vi "Trigger the captured image.vi"() -> ()   [LabVIEW 2018]
uses:
  LabViewDVPCamera/LabViewDVPCamera.lvlib
  <vilib>/picture/picture.llb/imagedata.ctl
panel:
  in  "image data":T1 caption="图像数据"
  in  "Trigger":bool
  in  "CloseFlg":i32
  out "handle":u32
  out "new picture":picture caption="新图片"
  in  "CameraList":u16(ring) items=["MGS130M-192.168.0.251"]
  in  "Set":bool
  in  "Close":bool
  in  "Open":bool
  in  "ScanCamera":bool
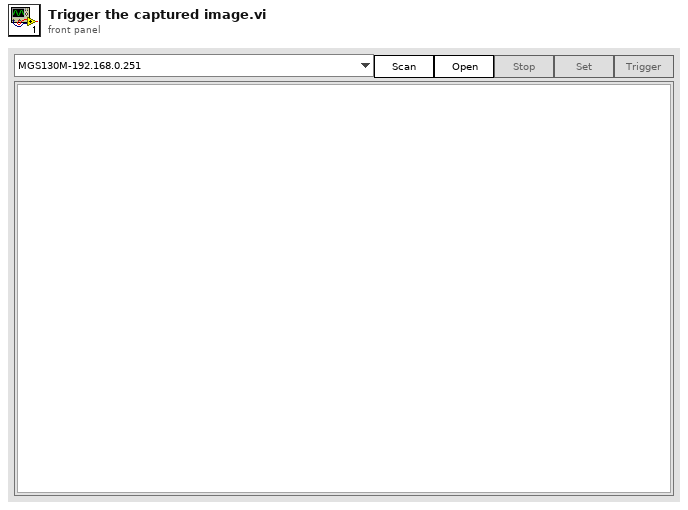
[diagram p1: front panel]
types:
  T1 = typedef "imagedata.ctl" = cluster{"image type":i32, "image depth":i32, "image":u8[], "mask":u8[], "colors":u32[], "Rectangle":cluster{"left":i16, "top":i16, "right":i16, "bottom":i16}}
  T2 = enum8{"Enabled", "Disabled", "Disabled and Grayed Out"}
  T3 = typedef "LVStringsAndValuesArrayTypeDef_U16.ctl" = cluster{"String":string, "Value":u16}[]
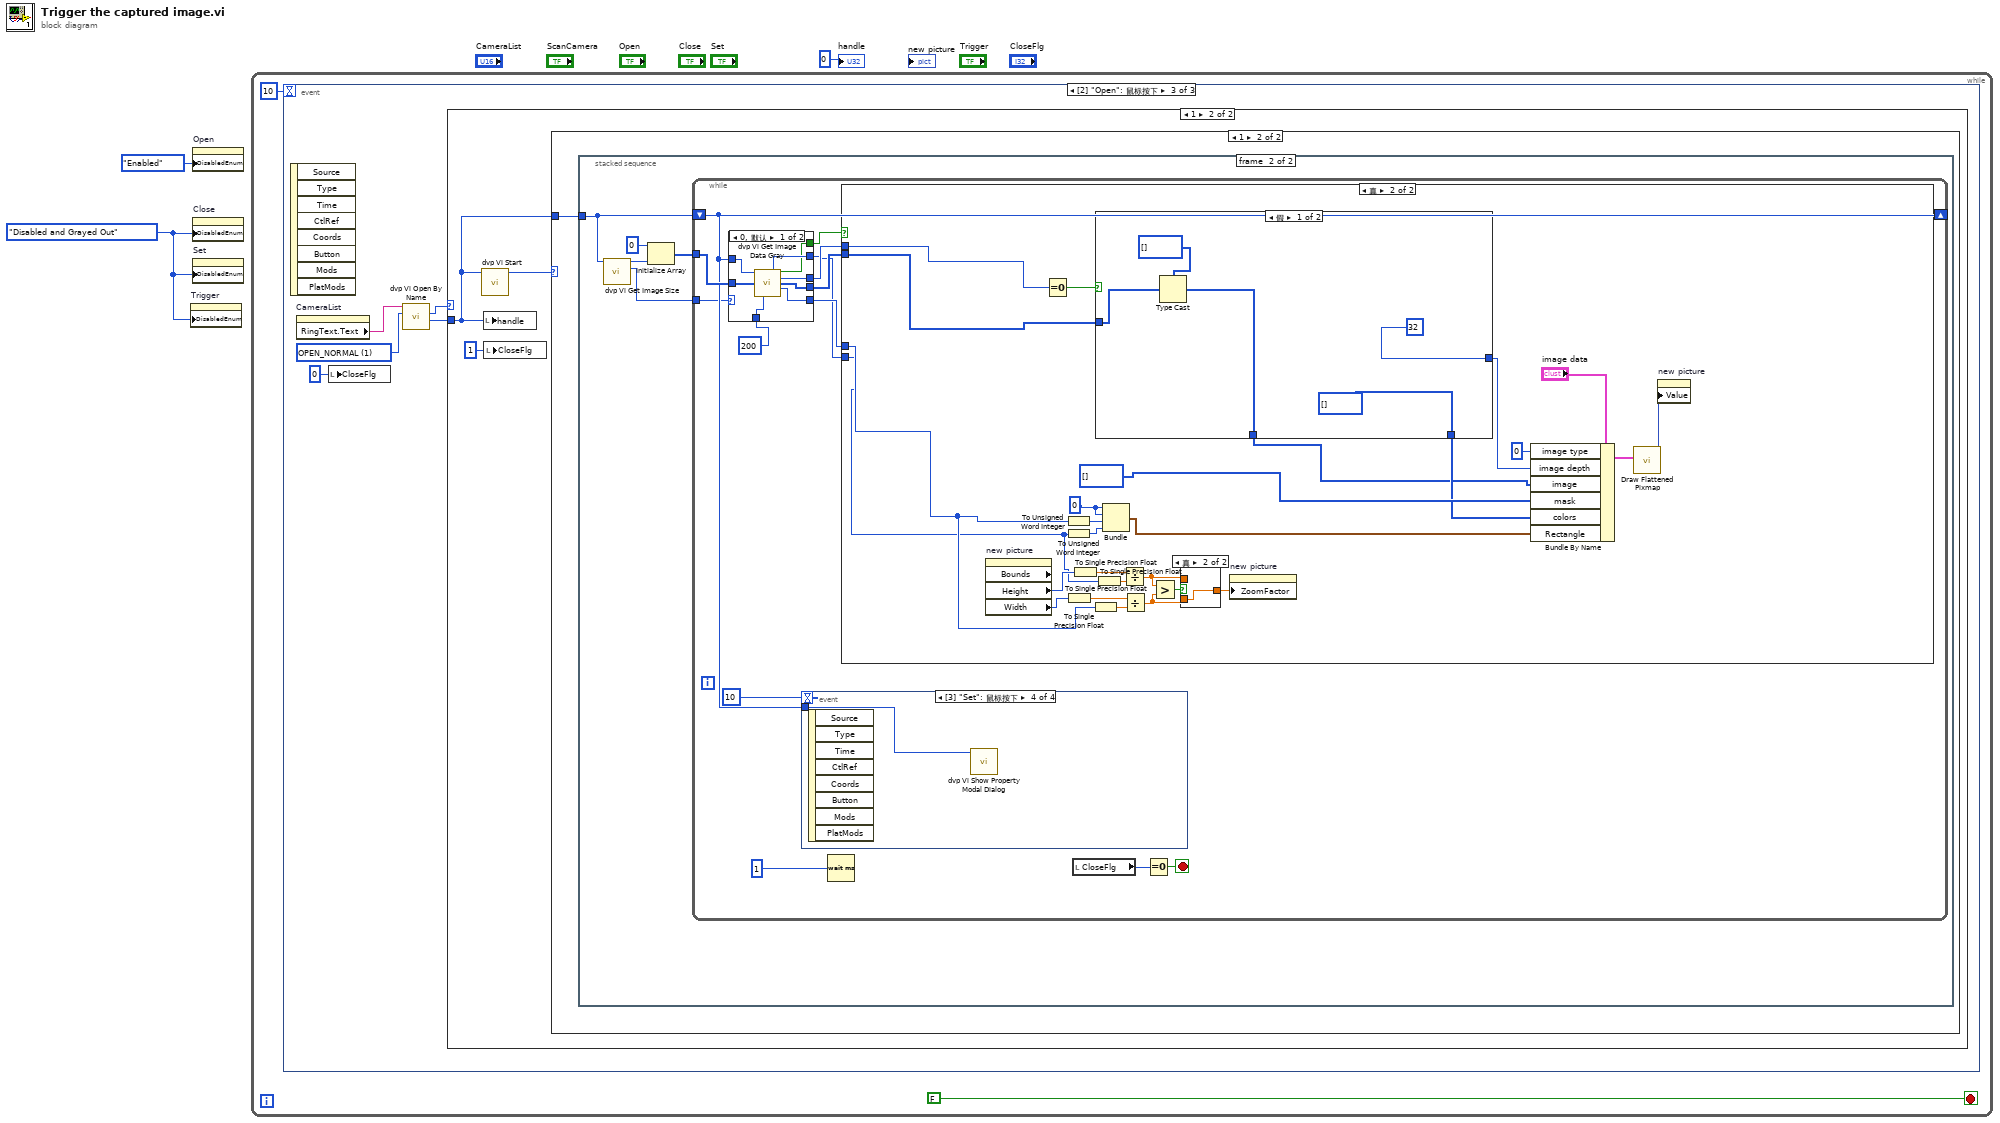
[diagram p0: block diagram]
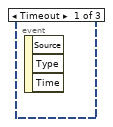
[diagram p2: hidden frame]
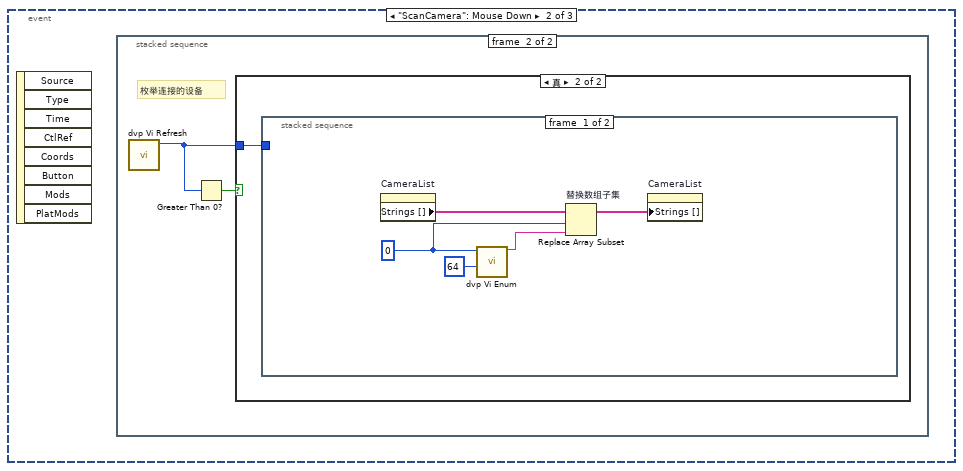
[diagram p3: hidden frame]
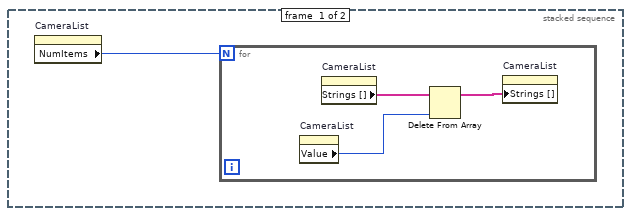
[diagram p4: hidden frame]
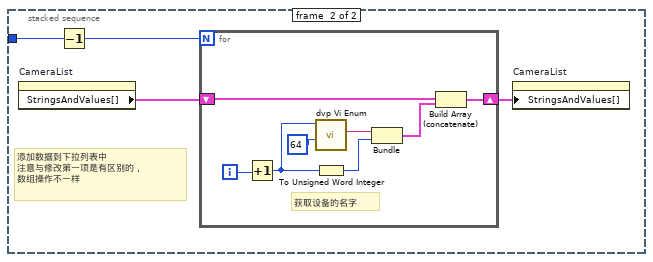
[diagram p6: hidden frame]
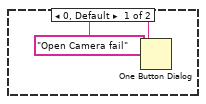
[diagram p7: hidden frame]
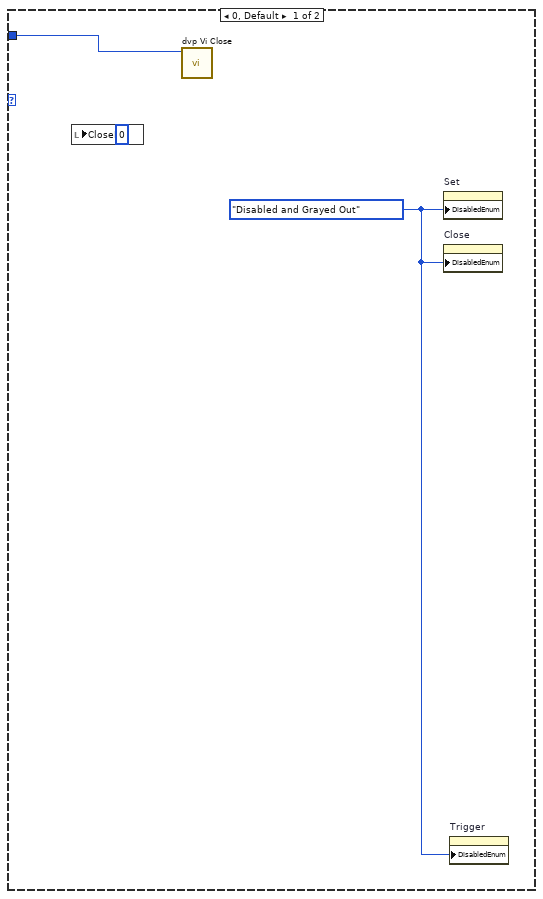
[diagram p8: hidden frame]
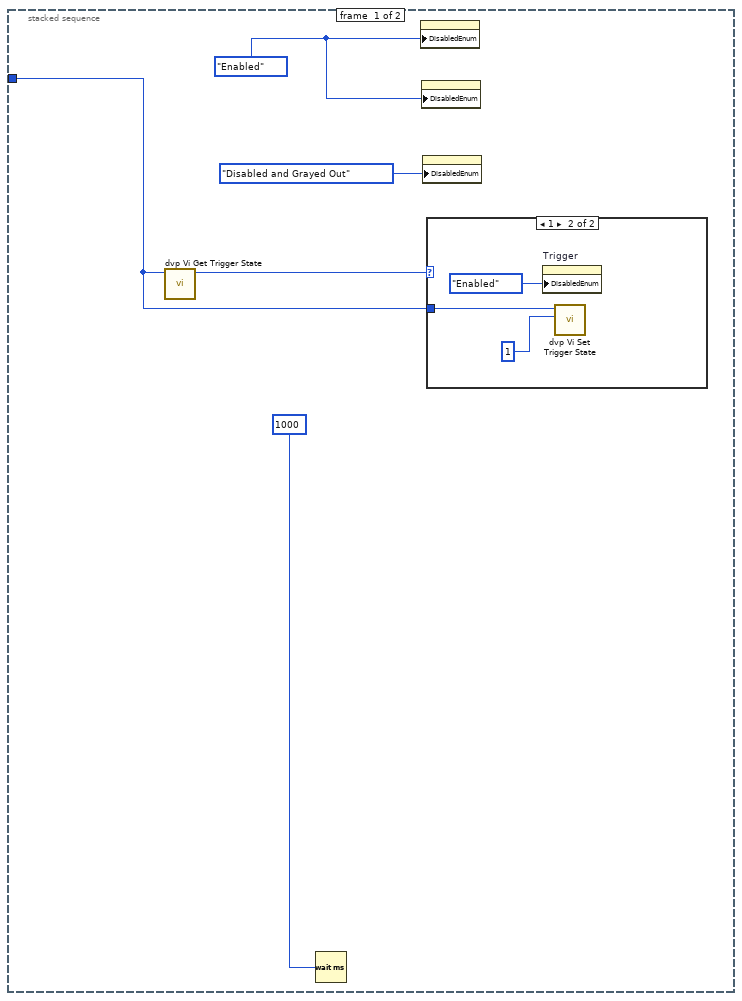
[diagram p9: hidden frame]
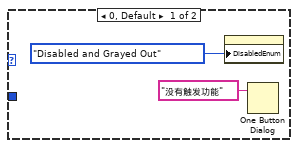
[diagram p10: hidden frame]
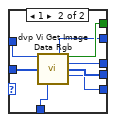
[diagram p11: hidden frame]
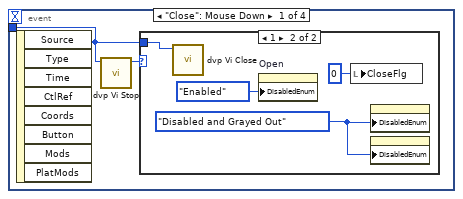
[diagram p12: hidden frame]
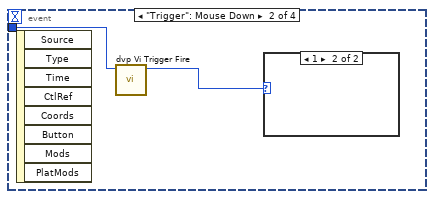
[diagram p14: hidden frame]
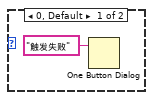
[diagram p15: hidden frame]
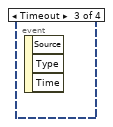
[diagram p16: hidden frame]
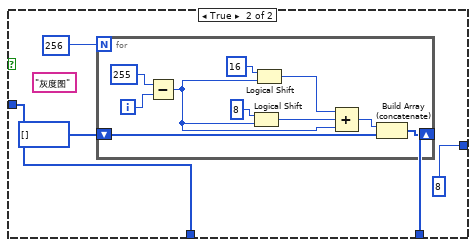
[diagram p19: hidden frame]
diagram:
  w1 = T2."Disabled and Grayed Out" ("禁用")
  n1 = property on="Trigger" class="Bool"("DisabledEnum"=w1) -> ()  [unwired: 2 in, 2 out]
  n2 = property on="Open" class="Bool"("DisabledEnum"=T2."Enabled" ("禁用")) -> ()  [unwired: 2 in, 2 out]
  n3 = property on="Close" class="Bool"("DisabledEnum"=w1) -> ()  [unwired: 2 in, 2 out]
  n4 = property on="Set" class="Bool"("DisabledEnum"=w1) -> ()  [unwired: 2 in, 2 out]
  n5 = while {
    stop <- FALSE stop-if-true
    n6 = event shown="[2] \"Open\": 鼠标按下" {
      selector: _ -> [_ _ _]
      dyn-events: _ -> [_ _ _]
      timeout: 10 -> [_ _ _]
      event Timeout {
        n7 = event-data() -> ()  [unwired: 1 in, 3 out]
      }
      event "ScanCamera": Mouse Down {
        n8 = event-data() -> ()  [unwired: 1 in, 8 out]
        n9 = stacked-sequence "清除下拉列表的数据" {
          frame #0 {
            n10 = property on="CameraList" class="Ring (严格)"() -> ("NumItems"=w6:u32)  [unwired: 2 in, 2 out]
            n11 = for {
              N: w6 -> [_]
              n12 = property on="CameraList" class="Ring (严格)"() -> ("Value"=w8:u16)  [unwired: 2 in, 2 out]
              n13 = property on="CameraList" class="Ring (严格)"() -> ("Strings []"=w7:string[])  [unwired: 2 in, 2 out]
              n14 = Delete From Array ("删除数组元素")(array=w7, index=w8) -> (array with subset deleted=w9:string[])  [unwired: 1 in, 1 out]
              n15 = property on="CameraList" class="Ring (严格)"("Strings []"=w9) -> ()  [unwired: 2 in, 2 out]
            }
          }
          frame #1 {
            # "枚举连接的设备"
            n16 = call "dvp Vi Refresh.vi"() -> ("pCount out"=w11:u32)  [unwired: 10 in, 1 out]
            n17 = Greater Than 0?(x=w11) -> (x > 0?=w10:bool)
            n18 = case shown="真" w10 {
              tunnel: w11 -> [_ w12]
              frame False {
                # "没有连接的设备直接退出不处理"
              }
              frame True {
                n19 = stacked-sequence {
                  tunnel: w12 -> [_ w19]
                  frame #0 {
                    w13 = u32 0 ("index")
                    n20 = property on="CameraList" class="Ring (严格)"() -> ("Strings []"=w16:string[])  [unwired: 2 in, 2 out]
                    n21 = call "dvp Vi Enum.vi"("unSize"=u32 64, "index"=w13) -> ("friendlyName out"=w15:string)  [unwired: 8 in, 1 out]
                    n22 = Replace Array Subset "替换数组子集"(array=w16, new element=w15, index=w13) -> (w17:string[])
                    n23 = property on="CameraList" class="Ring (严格)"("Strings []"=w17) -> ()  [unwired: 2 in, 2 out]
                  }
                  frame #1 {
                    # "添加数据到下拉列表中\n注意与修改第一项是有区别的，\n数组操作不一样"
                    n24 = property on="CameraList" class="Ring (严格)"() -> ("StringsAndValues[]"=w21:T3)  [unwired: 2 in, 2 out]
                    n25 = Decrement(x=w19) -> (x-1=w18:u32)
                    n26 = for {
                      N: w18 -> [_]
                      shift-right: [w28] -> w20
                      shift-left: w21 -> [w26]
                      i -> [w23]
                      # "获取设备的名字"
                      n27 = Increment(x=w23) -> (x+1=w22:i32)
                      n28 = call "dvp Vi Enum.vi"("unSize"=u32 64, "index"=w22) -> ("friendlyName out"=w29:string)  [unwired: 8 in, 1 out]
                      n29 = To Unsigned Word Integer(number=w22) -> (unsigned 16bit integer=w25:u16)
                      n30 = Bundle("friendlyName out"=w29, w25) -> (w27:cluster{"friendlyName out":string, u16})  [unwired: 1 in]
                      n31 = Build Array (concatenate)(w26, w27) -> (w28:T3)
                    }
                    n32 = property on="CameraList" class="Ring (严格)"("StringsAndValues[]"=w20) -> ()  [unwired: 2 in, 2 out]
                  }
                }
              }
            }
          }
        }
      }
      event "Open": Mouse Down {
        w32 = u32 1 items=["OPEN_OFFLINE", "OPEN_NORMAL"] ("type")
        n33 = event-data() -> ()  [unwired: 1 in, 8 out]
        n34 = property on="CameraList" class="Ring (严格)"() -> ("RingText.Text"=w31:string)  [unwired: 2 in, 2 out]
        n35 = local write "CloseFlg"(0 ("CloseFlg")) -> ()
        n36 = call "dvp Vi Open By Name.vi"("type"=w32, "friendlyName"=w31) -> ("pHandle out"=w34:u32, "function return"=w33:u32)  [unwired: 7 in, 1 out]
        n37 = case shown="1" w33 {
          tunnel: w34 -> [_ w38]
          frame 0, Default {
            n38 = One Button Dialog(message="Open Camera fail" ("消息")) -> ()  [unwired: 1 in, 1 out]
          }
          frame 1 {
            n39 = call "dvp Vi Start.vi"("handle"=w38) -> ("function return"=w36:u32)  [unwired: 10 in]
            n40 = local write "handle"(w38) -> ()
            n41 = local write "CloseFlg"(1 ("CloseFlg")) -> ()
            n42 = case shown="1" w36 {
              tunnel: w38 -> [w41 w42]
              frame 0, Default {
                w39 = T2."Disabled and Grayed Out" ("禁用")
                n43 = local write "CloseFlg"(0 ("CloseFlg")) -> ()
                n44 = call "dvp Vi Close.vi"("handle"=w41) -> ()  [unwired: 10 in, 1 out]
                n45 = property on="Set" class="Bool"("DisabledEnum"=w39) -> ()  [unwired: 2 in, 2 out]
                n46 = property on="Close" class="Bool"("DisabledEnum"=w39) -> ()  [unwired: 2 in, 2 out]
                n47 = property on="Trigger" class="Bool"("DisabledEnum"=w39) -> ()  [unwired: 2 in, 2 out]
              }
              frame 1 {
                n48 = stacked-sequence {
                  tunnel: w42 -> [w44 w55]
                  frame #0 {
                    w46 = T2."Enabled" ("禁用")
                    n49 = call "dvp Vi Get Trigger State.vi"("handle"=w44) -> ("function return"=w45:u32)  [unwired: 9 in, 1 out]
                    n50 = Wait (ms)(milliseconds to wait=u32 1000 ("等待时间（毫秒）")) -> ()  [unwired: 1 out]
                    n51 = property on="Set" class="Bool"("DisabledEnum"=w46) -> ()  [unwired: 2 in, 2 out]
                    n52 = property on="Close" class="Bool"("DisabledEnum"=w46) -> ()  [unwired: 2 in, 2 out]
                    n53 = property on="Open" class="Bool"("DisabledEnum"=T2."Disabled and Grayed Out" ("禁用")) -> ()  [unwired: 2 in, 2 out]
                    n54 = case shown="1" w45 {
                      tunnel: w44 -> [_ w51]
                      frame 0, Default {
                        n55 = property on="Trigger" class="Bool"("DisabledEnum"=T2."Disabled and Grayed Out" ("禁用")) -> ()  [unwired: 2 in, 2 out]
                        n56 = One Button Dialog(message="没有触发功能" ("消息")) -> ()  [unwired: 1 in, 1 out]
                      }
                      frame 1 {
                        n57 = property on="Trigger" class="Bool"("DisabledEnum"=T2."Enabled" ("禁用")) -> ()  [unwired: 2 in, 2 out]
                        n58 = call "dvp Vi Set Trigger State.vi"("TriggerState"=1, "handle"=w51) -> ()  [unwired: 9 in, 1 out]
                      }
                    }
                  }
                  frame #1 {
                    n59 = call "dvp Vi Get Image Size.vi"("handle"=w55) -> ("pformat out"=w53:i32, "function return"=w56:u32)  [unwired: 9 in]
                    n60 = Initialize Array(u32 0 ("元素"), w56) -> (w54:u32[])
                    n61 = while {
                      shift-right: [w64] -> _
                      shift-left: w55 -> [w64]
                      tunnel: w54 -> [w65]
                      tunnel: w53 -> [w63]
                      stop <- w69 stop-if-true
                      n62 = case shown="0, 默认" w63 {
                        tunnel: w65 -> [w78 w86]
                        tunnel: w64 -> [w77 w85]
                        tunnel: [w73 w84] -> w58
                        tunnel: [w75 w83] -> w61
                        tunnel: [w74 w82] -> w62
                        tunnel: [w76 w81] -> w59
                        tunnel: [w72 w80] -> w60
                        tunnel: u32 200 ("timeout") -> [w71 w79]
                        frame 0, Default {
                          n63 = call "dvp Vi Get Image Data Gray.vi"("handle"=w77, "pbuffer"=w78, "timeout"=w71) -> ("piHeight out"=w76:i32, "function return"=w73:bool, "pformat out"=w74:i32, "pbuffer out"=w75:u8[], "piWidth out"=w72:i32)  [unwired: 8 in]
                        }
                        frame 1 {
                          n64 = call "dvp Vi Get Image Data Rgb.vi"("handle"=w85, "pbuffer"=w86, "timeout"=w79) -> ("piHeight out"=w81:i32, "function return"=w84:bool, "pformat out"=w82:i32, "pbuffer out"=w83:u32[], "piWidth out"=w80:i32)  [unwired: 8 in]
                        }
                      }
                      n65 = event shown="[3] \"Set\": 鼠标按下" {
                        selector: _ -> [_ _ _ _]
                        dyn-events: _ -> [_ _ _ _]
                        timeout: 10 -> [_ _ _ _]
                        tunnel: w64 -> [w87 w94 _ w96]
                        event "Close": Mouse Down {
                          n66 = event-data() -> ()  [unwired: 1 in, 8 out]
                          n67 = call "dvp Vi Stop.vi"("handle"=w87) -> ("function return"=w88:u32)  [unwired: 10 in]
                          n68 = case shown="1" w88 {
                            tunnel: w87 -> [_ w90]
                            frame 0, Default {
                            }
                            frame 1 {
                              w89 = T2."Disabled and Grayed Out" ("禁用")
                              n69 = call "dvp Vi Close.vi"("handle"=w90) -> ()  [unwired: 10 in, 1 out]
                              n70 = property on="Open" class="Bool"("DisabledEnum"=T2."Enabled" ("禁用")) -> ()  [unwired: 2 in, 2 out]
                              n71 = local write "CloseFlg"(0 ("CloseFlg")) -> ()
                              n72 = property on="Close" class="Bool"("DisabledEnum"=w89) -> ()  [unwired: 2 in, 2 out]
                              n73 = property on="Set" class="Bool"("DisabledEnum"=w89) -> ()  [unwired: 2 in, 2 out]
                            }
                          }
                        }
                        event "Trigger": Mouse Down {
                          n74 = event-data() -> ()  [unwired: 1 in, 8 out]
                          n75 = call "dvp Vi Trigger Fire.vi"("handle"=w94) -> ("function return"=w93:u32)  [unwired: 10 in]
                          n76 = case shown="1" w93 {
                            frame 0, Default {
                              n77 = One Button Dialog(message="触发失败" ("消息")) -> ()  [unwired: 1 in, 1 out]
                            }
                            frame 1 {
                            }
                          }
                        }
                        event Timeout {
                          n78 = event-data() -> ()  [unwired: 1 in, 3 out]
                        }
                        event "Set": Mouse Down {
                          n79 = event-data() -> ()  [unwired: 1 in, 8 out]
                          n80 = call "dvp Vi Show Property Modal Dialog.vi"("handle"=w96) -> ()  [unwired: 10 in, 1 out]
                        }
                      }
                      n81 = Wait (ms)(milliseconds to wait=u32 1 ("等待时间（毫秒）")) -> ()  [unwired: 1 out]
                      n82 = case shown="真" w58 {
                        tunnel: w60 -> [_ w100]
                        tunnel: w59 -> [_ w99]
                        tunnel: w61 -> [_ w98]
                        tunnel: w62 -> [_ w101]
                        frame False {
                        }
                        frame True {
                          w123 = u16 0
                          n83 = property on="new picture" class="Pict" props=["Bounds", "Height", "Width"]() -> ("Height"=w102:u32, "Width"=w103:u32)  [unwired: 2 in, 3 out]
                          n84 = Equal To 0?(x=w101) -> (x = 0?=w119:bool)
                          n85 = To Unsigned Word Integer(number=w100) -> (unsigned 16bit integer=w122:u16)
                          n86 = To Unsigned Word Integer(number=w99) -> (unsigned 16bit integer=w121:u16)
                          n87 = To Single Precision Float(number=w103) -> (single precision float=w110:sgl)
                          n88 = To Single Precision Float(number=w102) -> (single precision float=w104:sgl)
                          n89 = To Single Precision Float(number=w100) -> (single precision float=w106:sgl)
                          n90 = case shown="假" w119 {
                            tunnel: [32 u8 8 ("image depth")] -> w116
                            tunnel: [u32[] [] ("数组") w132] -> w114
                            tunnel: w98 -> [w128 w131]
                            tunnel: [w127 w131] -> w97
                            frame False {
                              n91 = Type Cast(type=u8[] [], x=w128) -> (*(type *) &x=w127:u8[])
                            }
                            frame True {
                              (unwired) "灰度图"
                              n92 = for {
                                N: 256 -> [_]
                                shift-right: [w140] -> w132
                                shift-left: i32[] [] ("数组") -> [w139]
                                i -> [w136]
                                n93 = Subtract(x=255, y=w136) -> (x-y=w137:i32)
                                n94 = Logical Shift(y=i16 8, x=w137) -> (x << y=w142:i32)
                                n95 = Logical Shift(y=16 ("x"), x=w137) -> (x << y=w143:i32)
                                n96 = Compound Arithmetic op=ADD(w143, w142, w137) -> (w141:i32)
                                n97 = Build Array (concatenate)(w141, w139) -> (w140:i32[])
                              }
                            }
                          }
                          n98 = To Single Precision Float(number=w99) -> (single precision float=w105:sgl)
                          n99 = Bundle ("图像尺寸")(w123, w123, w122, w121) -> (w113:cluster{u16, u16, u16, u16})  [unwired: 1 in]
                          n100 = Divide(x=w104, y=w105) -> (x/y=w108:sgl)
                          n101 = Divide(x=w110, y=w106) -> (x/y=w109:sgl)
                          n102 = Greater?(x=w108, y=w109) -> (0:w107:bool)
                          n103 = case shown="真" w107 {
                            tunnel: w108 -> [w124 _]
                            tunnel: w109 -> [_ w125]
                            tunnel: [w124 w125] -> w111
                            frame False {
                            }
                            frame True {
                            }
                          }
                          n104 = property on="new picture" class="Pict"("ZoomFactor"=w111) -> ()  [unwired: 2 in, 2 out]
                          n105 = Bundle By Name(cluster="image data", "image type"=0, "image depth"=w116, "image"=w97, "mask"=u8[] [] ("无符号8位数组"), "colors"=w114, "Rectangle"=w113) -> (w117:T1)
                          n106 = call <vilib>:"Draw Flattened Pixmap.vi"("image data"=w117) -> ("new picture"=w120:picture)  [unwired: 8 in]
                          n107 = property on="new picture" class="Pict"("Value"=w120) -> ()  [unwired: 2 in, 2 out]
                        }
                      }
                      n108 = local read "CloseFlg"() -> (w68:i32)
                      n109 = Equal To 0?(x=w68) -> (x = 0?=w69:bool)
                    }
                  }
                }
              }
            }
          }
        }
      }
    }
  }
  "handle" <- u32 0 ("handle")
